vi "Lissage de signal.vi"() -> ()   [LabVIEW 2018]
panel:
  in  "stop":bool
  out "Graphe déroulant":cluster{dbl, dbl, dbl}(graph)
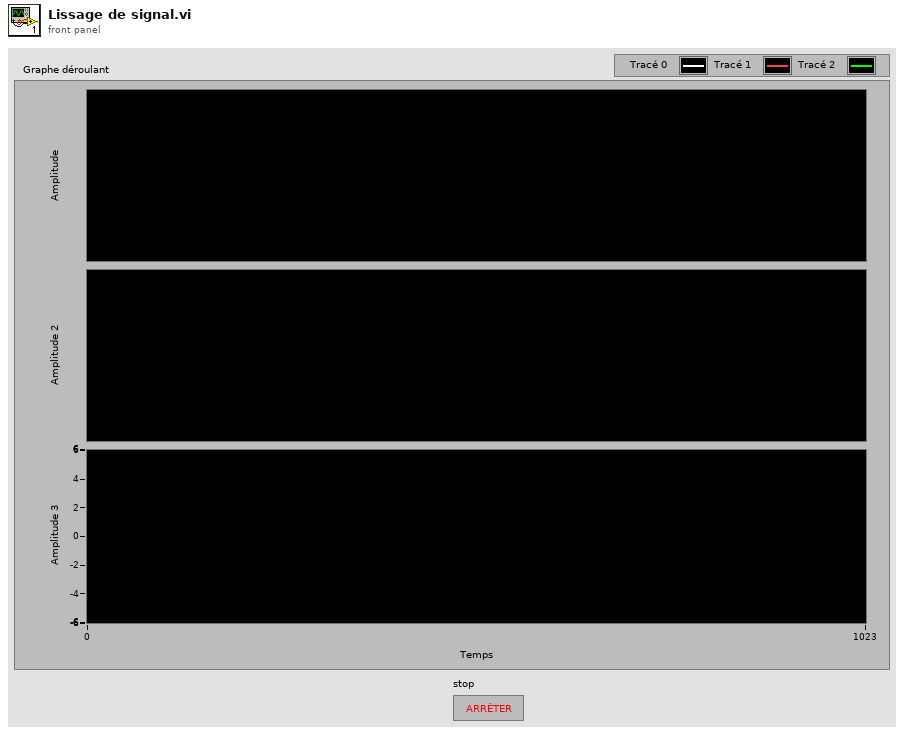
[diagram p1: front panel]
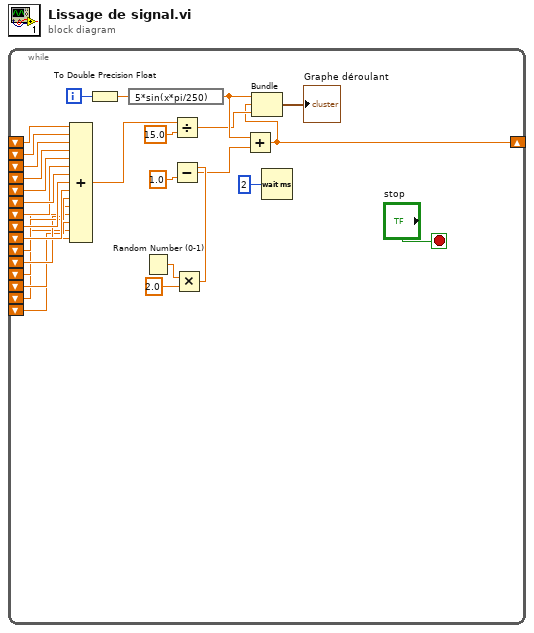
[diagram p0: block diagram]
diagram:
  n1 = while {
    shift-right: [w7] -> _
    shift-left: _ -> [w18]
    shift-left: _ -> [w17]
    shift-left: _ -> [w16]
    shift-left: _ -> [w15]
    shift-left: _ -> [w10]
    shift-left: _ -> [w14]
    shift-left: _ -> [w13]
    shift-left: _ -> [w11]
    shift-left: _ -> [w12]
    shift-left: _ -> [w5]
    shift-left: _ -> [w6]
    shift-left: _ -> [w2]
    shift-left: _ -> [w4]
    shift-left: _ -> [w3]
    shift-left: _ -> [w1]
    i -> [w19]
    stop <- "stop" stop-if-true
    n2 = Compound Arithmetic op=ADD(w18, w17, w16, w15, w14, w12, w13, w11, w10, w6, w5, w4, w3, w2, w1) -> (w9:dbl)
    n3 = To Double Precision Float(number=w19) -> (double precision float=w29:dbl)
    n4 = expression code="5*sin(x*pi/250)"(w29) -> (w21:dbl)
    n5 = Random Number (0-1)() -> (number: 0 to 1=w26:dbl)
    n6 = Divide(x=w9, y=15.0 ("x/y")) -> (x/y=w8:dbl)
    n7 = Multiply(x=w26, y=2.0) -> (x*y=w24:dbl)
    n8 = Subtract(x=w24, y=1.0) -> (x-y=w22:dbl)
    n9 = Add(x=w21, y=w22) -> (x+y=w7:dbl)
    n10 = Bundle(w21, w7, w8) -> (→"Graphe déroulant":cluster{dbl, dbl, dbl})  [unwired: 1 in]
    n11 = Wait (ms)(milliseconds to wait=u32 2 ("attente (ms)")) -> ()  [unwired: 1 out]
  }
